vi "Impulse Position Size.vi"(1 "Impulse Positions":T2(array[cluster])) -> (0 "Impulse Position size":i32[][](array[numeric]))   [LabVIEW 2016]
uses:
  type-defs/TD_Impulse Planes.ctl
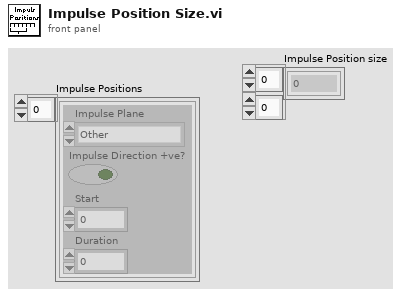
[diagram p1: front panel]
types:
  T1 = typedef "TD_Impulse Planes.ctl" = enum16{"Other", "Yaw", "Pitch", "Roll", "LARP", "RALP"}
  T2 = cluster{"Impulse Plane":T1, "Impulse Direction +ve?":bool, "Start":i32, "Duration":i32}[]
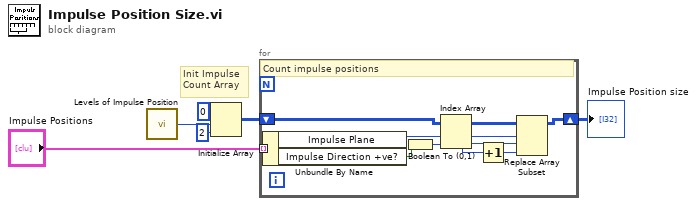
[diagram p0: block diagram]
diagram:
  # "Init Impulse\nCount Array"
  n1 = call "Levels of Impulse Position.vi"() -> ("Size"=w6:i32)  [unwired: 1 in]
  n2 = Initialize Array(0, w6, 2 ("dimension size")) -> (w5:i32[][])
  n3 = for {
    tunnel: "Impulse Positions" -> [w14] mode=indexing
    shift-right: [w7] -> w1
    shift-left: w5 -> [w13]
    # "Count impulse positions"
    n4 = Unbundle By Name(w14) -> ("Impulse Plane"=w11:T1, "Impulse Direction +ve?"=w12:bool)
    n5 = Boolean To (0,1)(Boolean=w12) -> (0, 1=w10:i16)
    n6 = Index Array(array=w13, index (row)=w11, index (col)=w10) -> (element=w8:i32)
    n7 = Increment(x=w8) -> (x+1=w9:i32)
    n8 = Replace Array Subset(array=w13, new element=w9, index (row)=w11, index (col)=w10) -> (w7:i32[][])
  }
  "Impulse Position size" <- w1
